vi "SLSC Calibrate UEGO.vi"(7 "settings.SLSC":T2={"SPI PHY Settings"={"Divide Value"=20, "Transfer Length (bits)"=32, "CS Asserted Polarity"=FALSE, "Clock Polarity (CPOL)"=FALSE, "Clock Phase (CPHA)"=FALSE, "Lengthen MISO Setup"=FALSE, "Direction Change Bit"=0, "MOSI Starts as Output"=FALSE, "Tristatable MOSI"=FALSE}, "Sample Rate (S/s)"=10000} {"SPI PHY Settings"."Direction Change Bit" max=64 step=1; "SPI PHY Settings"."Transfer Length (bits)" min=1 max=64 step=1}, 8 "Calibrate?":refnum<k21>="Calibration?", 9 "CS Bits":T6={"CS Bit 1"="Connector0/DIO0", "CS Bit 2"="Connector0/DIO0", "CS Bit 3"="Connector0/DIO0", "CS Bit 4"="Connector0/DIO0"}, 10 "SPI DIO Lines":T4={"SCLK"="Port0/DIO3", "MISO"="Port0/DIO3", "MOSI"="Port0/DIO3", "CS 0"="Port0/DIO3", "CS 1"="Port0/DIO4", "CS 2"="Port0/DIO4", "CS 3"="Port0/DIO1", "CS 4"="Port0/DIO4", "CS 5"="Port0/DIO4"}, 11 "slsc.calibration":T5) -> (3 "Complete?":T1)   [LabVIEW 2014, in "SLSC FPGA Toolkit.lvlib"]
uses:
  SLSC FPGA Toolkit.lvlib
  <vilib>/eio/EIONode/EIONode.xnode
  <vilib>/rvi/DataTransferAndStorage/Container/XNode/niFpgaContainer.xnode
  <vilib>/rvi/DataTransferAndStorage/Register/Emulation/niFpgaRegisterEmulationRefIn.vi
  <vilib>/Platform/TimedLoop/XDataNode/XDataNode.xnode
  <vilib>/Platform/TimedLoop/XDataNode/nitl_modes.ctl
  <vilib>/Platform/TimedLoop/XDataNode/XDNodeRunTimeDep.lvlib
  <vilib>/Platform/TimedLoop/XDataNode/wakeup.ctl
  <vilib>/Platform/TimedLoop/XDataNode/timing_clust.ctl
  SLSC Calibration Complete.ctl
  <vilib>/rvi/eio/common/nirviEmuTemplateMethod_errors.vi
  CD/Source/Shared/SPI Utility/CS Bits.ctl
  CD/Source/Shared/SLSC configuration Shared.lvlib
  <userlib>/_NI SPI IP/FPGA/Controllers/Public/Transfer Settings.ctl
  <userlib>/_NI SPI IP/FPGA/Controllers/NI SPI IP FPGA.lvlib
  <vilib>/SPI API/SPIAPI/DIO/SPI Digital IO Lines.ctl
  SLSC FPGA Inputs.ctl
  SLSC UEGO Calibration.ctl
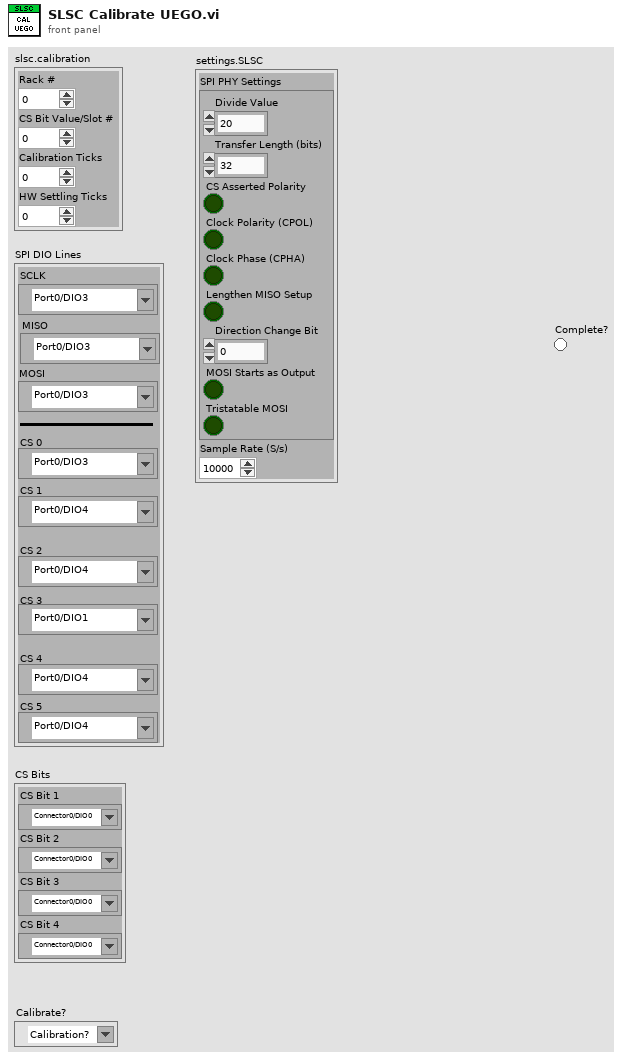
[diagram p1: front panel]
types:
  T1 = typedef "SLSC FPGA Toolkit.lvlib/SLSC Calibration Complete.ctl" = bool
  T2 = typedef "SLSC FPGA Toolkit.lvlib/SLSC FPGA Inputs.ctl" = cluster{"SPI PHY Settings":T3, "Sample Rate (S/s)":u32}
  T3 = typedef "NI SPI IP FPGA.lvlib/Transfer Settings.ctl" = cluster{"Divide Value":u8, "Transfer Length (bits)":u8, "CS Asserted Polarity":bool, "Clock Polarity (CPOL)":bool, "Clock Phase (CPHA)":bool, "Lengthen MISO Setup":bool, "Direction Change Bit":u8, "MOSI Starts as Output":bool, "Tristatable MOSI":bool}
  T4 = typedef "SPI Digital IO Lines.ctl" = cluster{"SCLK":refnum<k21>, "MISO":refnum<k21>, "MOSI":refnum<k21>, "CS 0":refnum<k21>, "CS 1":refnum<k21>, "CS 2":refnum<k21>, "CS 3":refnum<k21>, "CS 4":refnum<k21>, "CS 5":refnum<k21>}
  T5 = typedef "SLSC FPGA Toolkit.lvlib/SLSC UEGO Calibration.ctl" = cluster{"Rack #":u8, "CS Bit Value/Slot #":u8, "Calibration Ticks":u32, "HW Settling Ticks":u32}
  T6 = typedef "SLSC configuration Shared.lvlib/CS Bits.ctl" = cluster{"CS Bit 1":refnum<k21>, "CS Bit 2":refnum<k21>, "CS Bit 3":refnum<k21>, "CS Bit 4":refnum<k21>}
  T7 = enum16{"Initialize", "Assert CS", "Starts Calibration", "Stops Calibration", "Deassert CS"}
  T8 = typedef "XDNodeRunTimeDep.lvlib/timing_clust.ctl" = cluster{"Expected End [f-1]":u64, "Actual End [f-1]":u64, "Finished Late? [f-1]":bool, "Expected End [i-1]":u64, "Actual End [i-1]":u64, "Finished Late? [i-1]":bool, "Expected Start [i]":u64, "Actual Start [i]":u64, "Expected Start [f]":u64, "Actual Start [f]":u64, "Source Name":string, "Structure Name":string, "Period":i64, "Deadline":i64, "Offset":i64, "Start":i64, "Priority":i32, "Timeout":i32, "Mode":T9, "Wakeup Reason":T10, "Error":errorcluster, "Source Type":string, "Secondary Source Type":string, "Global End Time":u64, "Global Start Time":u64, "Frame Duration":u64, "Iteration Duration":u64, "Assigned CPU":i32, "I/O Scan Engine Mode":u32}
  T9 = typedef "XDNodeRunTimeDep.lvlib/nitl_modes.ctl" = enum32{"No Change", "Process missed periods, maintain original phase", "Discard missed periods, maintain original phase", "Process missed periods, ignore original phase", "Discard missed periods, ignore original phase"}
  T10 = typedef "XDNodeRunTimeDep.lvlib/wakeup.ctl" = enum32{"Normal", "Aborted", "Asynchronous wakeup", "Timing source error", "Timed loop error", "Timeout"}
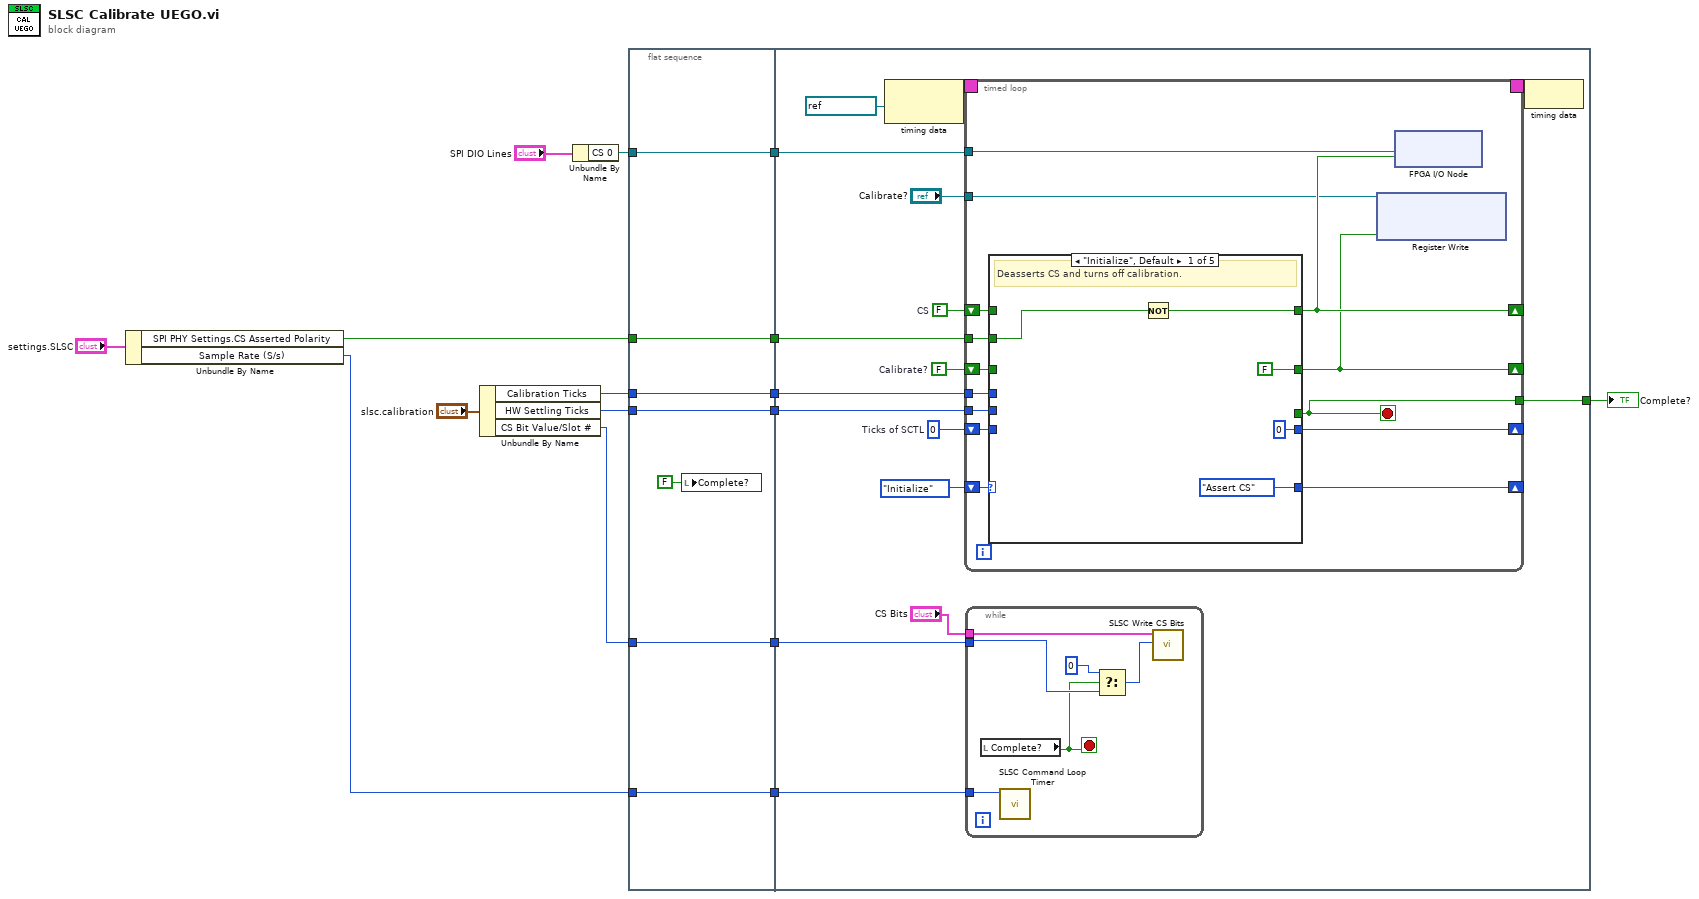
[diagram p0: block diagram]
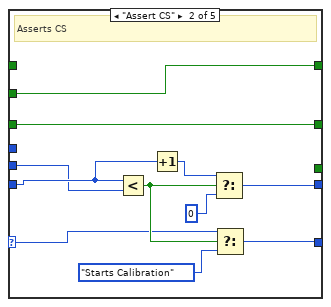
[diagram p2: hidden frame]
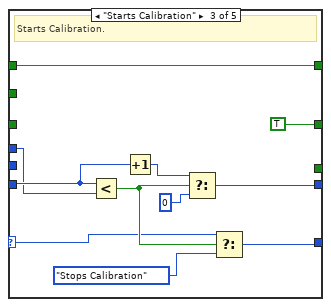
[diagram p3: hidden frame]
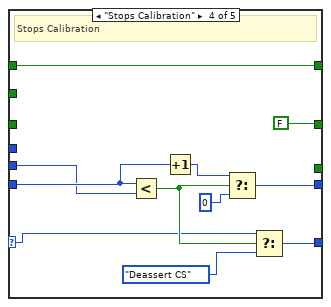
[diagram p4: hidden frame]
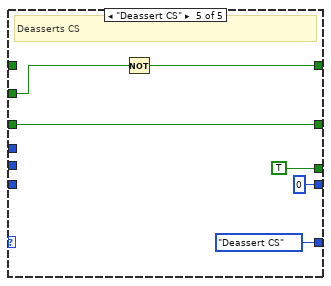
[diagram p5: hidden frame]
diagram:
  n1 = Unbundle By Name("settings.SLSC") -> ("SPI PHY Settings.CS Asserted Polarity"=w13:bool, "Sample Rate (S/s)"=w10:u32)
  n2 = Unbundle By Name("slsc.calibration") -> ("Calibration Ticks"=w9:u32, "HW Settling Ticks"=w8:u32, "CS Bit Value/Slot #"=w11:u8)
  n3 = Unbundle By Name("SPI DIO Lines") -> ("CS 0"=w15:refnum<k21>)
  n4 = flat-sequence {
    tunnel: w8 -> [w18]
    tunnel: w9 -> [w19]
    tunnel: w10 -> [w20]
    tunnel: w11 -> [w21]
    tunnel: w13 -> [w22]
    tunnel: w15 -> [w23]
    tunnel: [w23] -> w6
    tunnel: [w22] -> w5
    tunnel: [w21] -> w4
    tunnel: [w20] -> w3
    tunnel: [w19] -> w2
    tunnel: [w18] -> w1
    tunnel: [w24] -> w7
    tunnel: w6 -> [w35]
    tunnel: w5 -> [w34]
    tunnel: w4 -> [w29]
    tunnel: w3 -> [w28]
    tunnel: w2 -> [w27]
    tunnel: w1 -> [w26]
    frame #0 {
      n5 = local write "Complete?"(T1 FALSE ("Complete?")) -> ()
    }
    frame #1 {
      w25 = FALSE  # Calibrate?
      w31 = u32 0  # Ticks of SCTL
      w33 = FALSE  # CS
      n6 = node-c288(refnum<k21> "120MHz" ("Source Name")) -> (w39:T8)
      n7 = timed-loop {
        shift-right: [w57] -> _
        shift-left: T7."Initialize" -> [w59]
        tunnel: w35 -> [w55]
        tunnel: w34 -> [w58]
        tunnel: "Calibrate?" -> [w48]
        tunnel: [w56] -> w24
        shift-right: [w54] -> _
        shift-left: w33 -> [w53]
        timing: w39 -> [_]
        timing-out: [_] -> w38
        shift-right: [w49] -> _
        shift-left: w31 -> [w52]
        tunnel: w27 -> [w51]
        tunnel: w26 -> [w50]
        shift-right: [w47] -> _
        shift-left: w25 -> [w46]
        stop <- w56 stop-if-true
        n8 = case shown="\"Initialize\", Default" w59 {
          selector: w59 -> [_ w68 w80 w91 _]
          tunnel: [_ _ _ _ TRUE] -> w56
          tunnel: w58 -> [w64 w75 _ _ w102]
          tunnel: [T7."Assert CS" w66 w78 w89 T7."Deassert CS"] -> w57
          tunnel: [w62 w75 w86 w97 w100] -> w54
          tunnel: w53 -> [_ _ w86 w97 _]
          tunnel: w52 -> [_ w74 w82 w93 _]
          tunnel: w51 -> [_ _ w77 _ _]
          tunnel: w50 -> [_ w70 _ w92 _]
          tunnel: [u32 0 ("f") w71 w81 w88 u32 0 ("f")] -> w49
          tunnel: [FALSE ("Calibrate?") w65 TRUE ("Calibrate?") FALSE ("Calibrate?") w98] -> w47
          tunnel: w46 -> [_ w65 _ _ w98]
          frame "Initialize", Default {
            # "Deasserts CS and turns off calibration."
            n9 = Not(x=w64) -> (.not. x?=w62:bool)
          }
          frame "Assert CS" {
            # "Asserts CS"
            n10 = Less?(x=w74, y=w70) -> (x < y?=w69:bool)
            n11 = Increment(x=w74) -> (x+1=w73:u32)
            n12 = Select(t=w73, s=w69, f=u16 0) -> (s? t:f=w71:u32)
            n13 = Select(t=w68, s=w69, f=T7."Starts Calibration") -> (s? t:f=w66:T7)
          }
          frame "Starts Calibration" {
            # "Starts Calibration."
            n14 = Less?(x=w82, y=w77) -> (x < y?=w83:bool)
            n15 = Increment(x=w82) -> (x+1=w85:u32)
            n16 = Select(t=w85, s=w83, f=u16 0) -> (s? t:f=w81:u32)
            n17 = Select(t=w80, s=w83, f=T7."Stops Calibration") -> (s? t:f=w78:T7)
          }
          frame "Stops Calibration" {
            # "Stops Calibration"
            n18 = Less?(x=w93, y=w92) -> (x < y?=w94:bool)
            n19 = Increment(x=w93) -> (x+1=w96:u32)
            n20 = Select(t=w96, s=w94, f=u16 0) -> (s? t:f=w88:u32)
            n21 = Select(t=w91, s=w94, f=T7."Deassert CS") -> (s? t:f=w89:T7)
          }
          frame "Deassert CS" {
            # "Deasserts CS"
            n22 = Not(x=w102) -> (.not. x?=w100:bool)
          }
        }
        n23 = xnode ("Register Write")("Data"=w47, "Register In"=w48) -> ()  [unwired: 1 out]
        n24 = xnode "FPGA I/O Node"("I/O Item"=w54, "FPGA I/O In"=w55) -> ()  [unwired: 1 out]
      }
      n25 = while {
        tunnel: "CS Bits" -> [w45]
        tunnel: w29 -> [w42]
        tunnel: w28 -> [w44]
        stop <- w40 stop-if-true
        n26 = local read "Complete?"() -> (w40:T1)
        n27 = call "SLSC Command Loop Timer.vi"("inputs.Sample Rate (S/s)"=w44) -> ()  [unwired: 8 in, 3 out]
        n28 = Select(t=u8 0, s=w40, f=w42) -> (s? t:f=w41:u8)
        n29 = call "SLSC Write CS Bits.vi"("CS Bit Value/Slot #"=w41, "CS Bits"=w45) -> ()  [unwired: 10 in]
      }
      n30 = node-c288(w38) -> ()
    }
  }
  "Complete?" <- w7
